vi "XY Graph Get Selected Plot Index.vi"(8 "error in (no error)":errorcluster, 11 "Selected Plot Info":T1) -> (0 "error out":errorcluster, 2 "Plot at Coordinates":i32, 3 "XYGraph out":T2, 4 "Plot Index in (dup)":i32)   [LabVIEW 2021, in "XY Graph Add-Ons.lvlib"]
uses:
  XY Graph Refnum.ctl
  XY Graph Selected Plot Info.ctl
  <vilib>/Utility/miscctls.llb/LVPoint32TypeDef.ctl
  Get Plot at Mouse Click (XY Graph)/Get Plot at Mouse Click [AAC].vi
  XY Graph Add-Ons.lvlib
  Graphs.lvlib
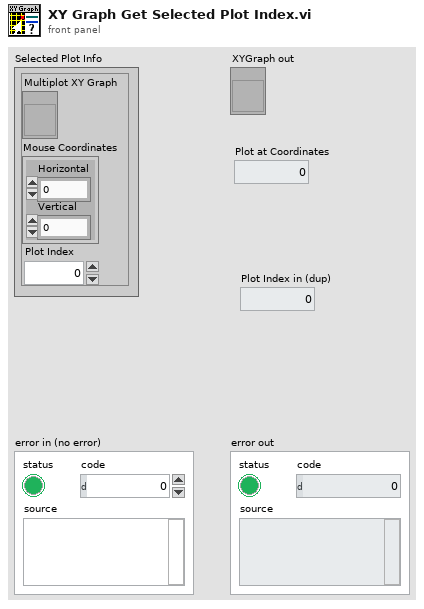
[diagram p1: front panel]
types:
  T1 = typedef "XY Graph Add-Ons.lvlib/XY Graph Selected Plot Info.ctl" = cluster{"Multiplot XY Graph":T2, "Mouse Coordinates":T3, "Plot Index":i32}
  T2 = typedef "XY Graph Add-Ons.lvlib/XY Graph Refnum.ctl" = refnum<vi>
  T3 = typedef "LVPoint32TypeDef.ctl" = cluster{"Horizontal":i32, "Vertical":i32}
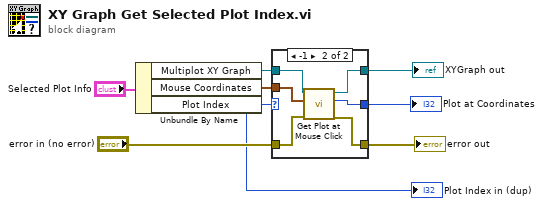
[diagram p0: block diagram]
diagram:
  n1 = Unbundle By Name("Selected Plot Info") -> ("Multiplot XY Graph"=w4:T2, "Mouse Coordinates"=w3:T3, "Plot Index"=w2:i32)
  "Plot Index in (dup)" <- w2
  n2 = case shown="-1" w2 {
    selector: w2 -> [w9 _]
    tunnel: w4 -> [w11 w17]
    tunnel: w3 -> [_ w16]
    tunnel: "error in (no error)" -> [w10 w15]
    tunnel: [w11 w14] -> w8
    tunnel: [w10 w13] -> w7
    tunnel: [w9 w12] -> w1
    frame 0, Default {
    }
    frame -1 {
      n3 = call-poly "Get Plot at Mouse Click.vi"("error in (no error)"=w15, "Mouse Click Coordinates"=w16, "XYGraph Ref"=w17) -> ("error out"=w13:errorcluster, "Plot at Coordinates"=w12:i32, "XYGraph Ref"=w14:T2)  [unwired: 2 in, 4 out]
    }
  }
  "XYGraph out" <- w8
  "error out" <- w7
  "Plot at Coordinates" <- w1
